vi "1DTo2D.vi"(8 "error in (no error)":errorcluster, 11 "reshapeInfo":T1) -> (0 "error in (no error) 2":errorcluster, 3 "Array out":i16[][](array[numeric]))   [LabVIEW 2011]
uses:
  reshapeINfo_TypDef.ctl
  emptyArray_TYpDEf.ctl
  emptyArrayCamX_TypDef.ctl
  reshapeArrayCommand_TypDEf.ctl
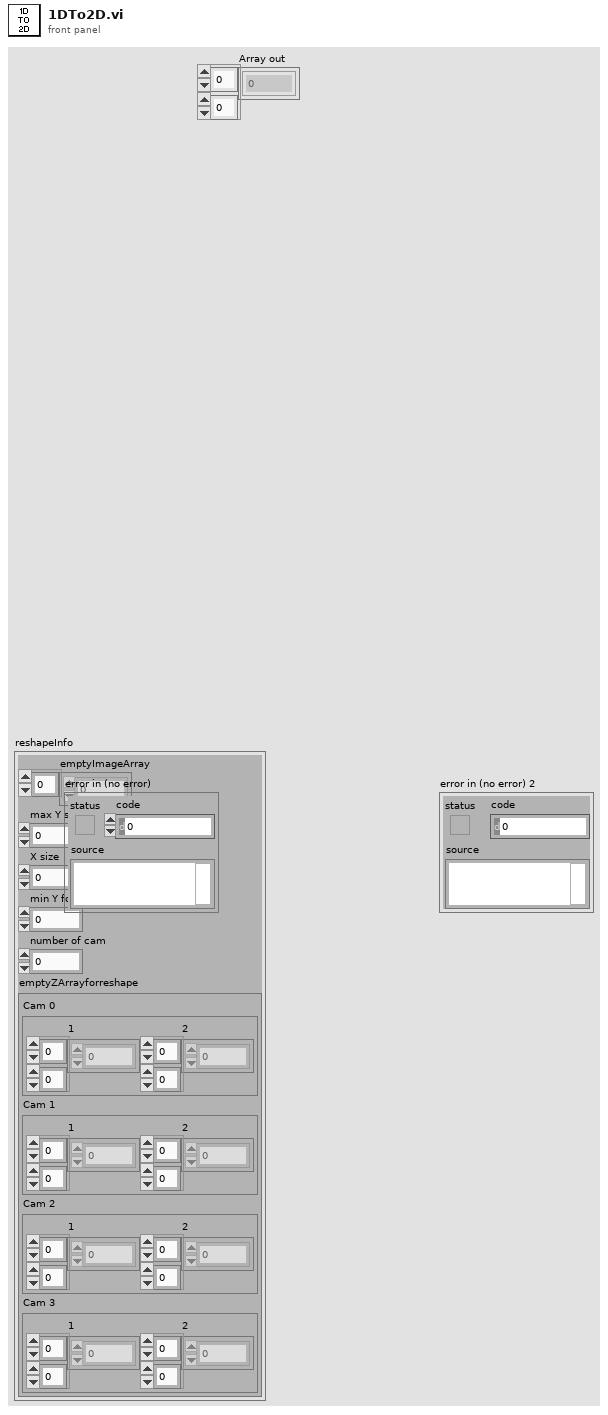
[diagram p1: front panel]
types:
  T1 = typedef "reshapeINfo_TypDef.ctl" = cluster{"emptyImageArray":dbl[], "max Y size":i32, "X size":i32, "min Y for allImage":dbl, "number of cam":i32, "emptyZArrayforreshape":T2}
  T2 = typedef "emptyArray_TYpDEf.ctl" = cluster{"Cam 0":T3, "Cam 1":T3, "Cam 2":T3, "Cam 3":T3}
  T3 = typedef "emptyArrayCamX_TypDef.ctl" = cluster{"1":dbl[][], "2":dbl[][]}
  T4 = typedef "reshapeArrayCommand_TypDEf.ctl" = enum16{"init array", "addImage", "read", "init resolution"}
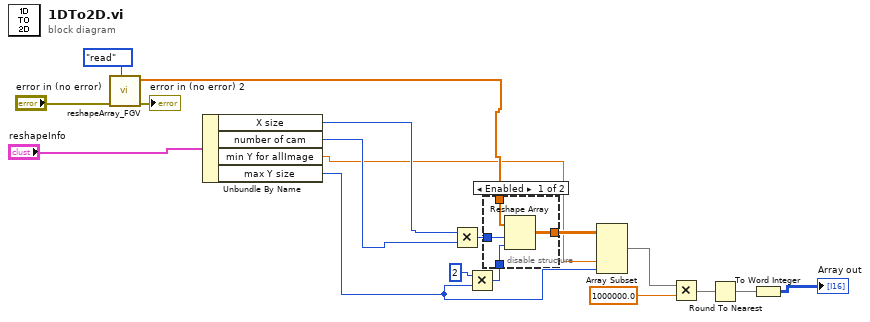
[diagram p0: block diagram]
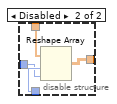
[diagram p2: hidden frame]
diagram:
  n1 = call "reshapeArray_FGV.vi"("command"=reshapeArrayCommand_TypDEf."read", "error in (no error)"="error in (no error)") -> ("error in (no error) 2"=→"error in (no error) 2":errorcluster, "ImageArray"=w11:dbl[])  [unwired: 8 in]
  n2 = Unbundle By Name("reshapeInfo") -> ("X size"=w14:i32, "number of cam"=w13:i32, "min Y for allImage"=w7:dbl, "max Y size"=w6:i32)
  n3 = Multiply(x=w14, y=w13) -> (x*y=w16:i32)
  n4 = Multiply(x=2 ("length"), y=w6) -> (x*y=w17:i32)
  n5 = disable-structure shown="Enabled" {
    disable-tunnel: [w22 w23] -> w8
    disable-tunnel: w17 -> [w21 w25]
    disable-tunnel: w16 -> [w20 w24]
    disable-tunnel: w11 -> [w19 w26]
    frame Enabled {
      n6 = Reshape Array(w19, w20, w21) -> (w22:dbl[][])
    }
    frame Disabled {
      n7 = Reshape Array(w26, w25, w24) -> (w23:dbl[][])
    }
  }
  n8 = Array Subset(array=w8, index (col)=w7, length (col)=w6) -> (w5:dbl[][])  [unwired: 2 in]
  n9 = Multiply(x=w5, y=1000000.0) -> (x*y=w3:dbl[][])
  n10 = Round To Nearest(number=w3) -> (nearest integer value=w2:dbl[][])
  n11 = To Word Integer(number=w2) -> (16bit integer=→"Array out":i16[][])
